vi "AddTagBusWebServiceToProject.vi"() -> ()   [LabVIEW 2013]
uses:
  <resource>/Framework/Providers/ws_project_provider/common/NI Web Service Provider.lvlib
panel:
  out "error out":errorcluster
  # "Please wait..."
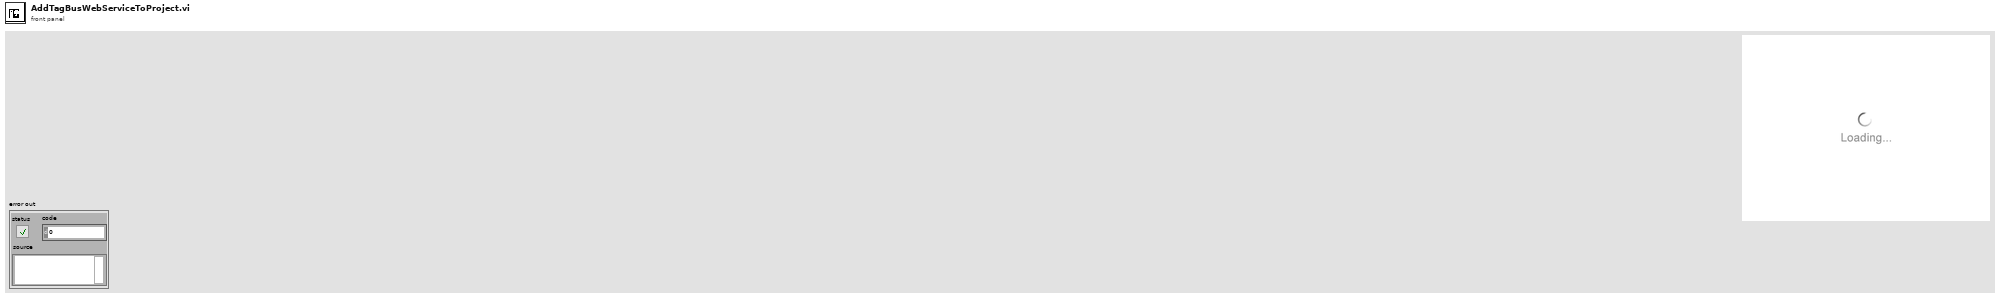
[diagram p1: front panel]
types:
  T1 = typedef "ws.ctl" = cluster{"Web Service":T2, "startup":path[], "wsmethods":path[], "private content":path[], "public content":path[], "wm ids":string[]}
  T2 = typedef "NI Web Service Provider.lvlib/Web Service.ctl" = cluster{"Name":string, "GUID":string, "Version":cluster{"Major":u16, "Minor":u16, "Fix":u16, "Build":u16}, "Serve index.html":bool, "Remote debugging":bool, "SSE2 optimizations":bool, "Exclusions":cluster{"Disconnect type definitions":bool, "Remove unused polymorphic VI instances":bool, "Remove unused members of project libraries":bool, "Modify project library file after removing unused members":bool}, "Disconnect inline subVIs":bool, "Auto-increment version":bool, "Web service VIs":T3[], "Static Permissions":string}
  T3 = typedef "NI Web Service Provider.lvlib/Web Service VI.ctl" = cluster{"item":u64, "item ID":string, "Web Service VI Type":T4, "Method":T5, "Load at startup":bool, "Keep in memory":bool, "Output type":T6, "Output format":T7, "Use headers":bool, "Buffered":bool, "Require API key":bool, "Permissions":string, "Standard URL":bool, "Include VI name in URL":bool, "Custom URL":string}
  T4 = typedef "NI Web Service Provider.lvlib/Web Service VI Type.ctl" = enum16{"<DUMMY>", "Web Method", "Auxiliary", "Internal", "Content"}
  T5 = typedef "NI Web Service Provider.lvlib/Web Service VI Method.ctl" = enum16{"<DUMMY>", "GET", "PUT", "POST", "DELETE", "OPTIONS", "HEAD", "TRACE"}
  T6 = typedef "NI Web Service Provider.lvlib/Web Service VI Output Type.ctl" = enum16{"Terminal", "Stream"}
  T7 = typedef "NI Web Service Provider.lvlib/Web Service VI Output Format.ctl" = enum16{"<DUMMY>", "Text", "XML", "HTML", "JSON"}
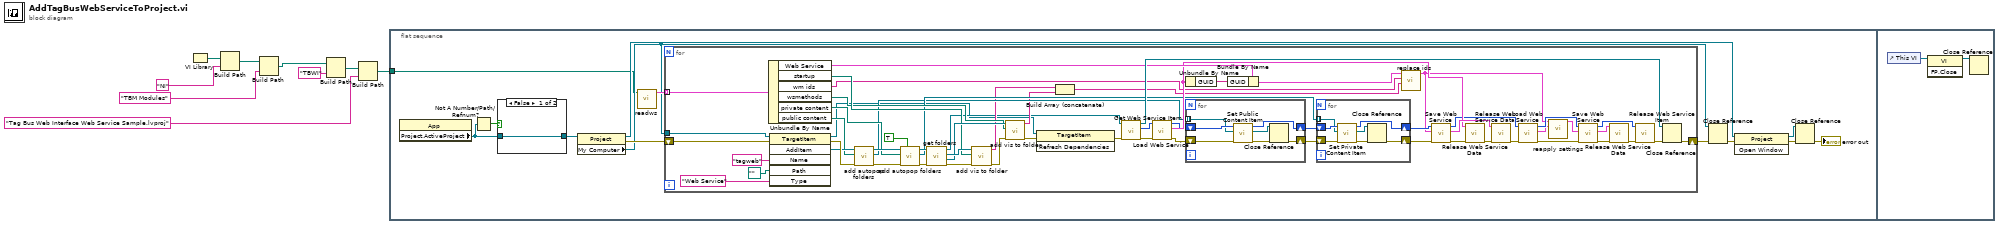
[diagram p0: block diagram]
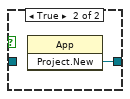
[diagram p2: hidden frame]
diagram:
  n1 = VI Library() -> (path=w5:path)
  n2 = Build Path(base path=w5, name or relative path="NI") -> (appended path=w7:path)
  n3 = Build Path(base path=w7, name or relative path="TBM Modules") -> (appended path=w4:path)
  n4 = Build Path(base path=w4, name or relative path="TBWI") -> (appended path=w3:path)
  n5 = Build Path(base path=w3, name or relative path="Tag Bus Web Interface Web Service Sample.lvproj") -> (appended path=w1:path)
  n6 = flat-sequence {
    tunnel: w1 -> [w10]
    frame #0 {
      n7 = property class="App"() -> ("Project.ActiveProject"=w13:refnum<vi>)  [unwired: 2 in, 2 out]
      n8 = Not A Number/Path/Refnum?(number/path/refnum=w13) -> (NaN/Path/Refnum?=w12:bool)
      n9 = case shown="False" w12 {
        tunnel: [w23 w24] -> w11
        tunnel: w13 -> [w23 _]
        frame False {
        }
        frame True {
          n10 = invoke class="App" method="Project.New"() -> ("Project:New"=w24:refnum<vi>)  [unwired: 3 in, 2 out]
        }
      }
      n11 = property class="Project"(reference=w11) -> (reference out=w19:refnum<vi>, error out=w21:errorcluster, "My Computer"=w15:refnum<vi>)  [unwired: 1 in]
      n12 = call "readws.vi"("Path"=w10) -> ("Array"=w22:T1[])  [unwired: 9 in, 1 out]
      n13 = for {
        tunnel: w22 -> [w66] mode=indexing
        shift-right: [w78] -> w14
        shift-left: w21 -> [w77]
        tunnel: w15 -> [w29]
        n14 = Unbundle By Name(w66) -> ("Web Service"=w61:T2, "startup"=w63:path[], "wm ids"=w44:string[], "wsmethods"=w62:path[], "private content"=w64:path[], "public content"=w65:path[])
        n15 = invoke class="TargetItem" method="AddItem"(reference=w29, error in=w77, "Name"="tagweb", "Path"=path "", "Type"="Web Service") -> (reference out=w25:refnum<vi>, error out=w76:errorcluster, "AddItem"=w75:refnum<vi>)  [unwired: 1 in, 3 out]
        n16 = call "add autopop folders.vi"("error in (no error)"=w76, "autopop"=w65, "ProjectItem in"=w75) -> ("error out"=w70:errorcluster, "items out"=w47:refnum<vi>[], "ProjectItem out"=w67:refnum<vi>)  [unwired: 6 in]
        n17 = call "add autopop folders.vi"("private?"=TRUE, "error in (no error)"=w70, "autopop"=w64, "ProjectItem in"=w67) -> ("error out"=w69:errorcluster, "items out"=w48:refnum<vi>[], "ProjectItem out"=w68:refnum<vi>)  [unwired: 5 in]
        n18 = call "get folders.vi"("error in"=w69, "web service in"=w68) -> ("error out"=w73:errorcluster, "web methods"=w72:refnum<vi>, "startup"=w74:refnum<vi>, "Web service project item out"=w26:refnum<vi>)  [unwired: 6 in]
        n19 = call "add vis to folder.vi"("error in"=w73, "startup"=w63, "ProjectItem in"=w74) -> ("error out"=w71:errorcluster, "ids"=w41:string[])  [unwired: 7 in]
        n20 = call "add vis to folder.vi"("error in"=w71, "startup"=w62, "ProjectItem in"=w72) -> ("error out"=w28:errorcluster, "ids"=w43:string[])  [unwired: 7 in]
        n21 = invoke class="TargetItem" method="Refresh Dependencies"(reference=w25, error in=w28) -> (error out=w27:errorcluster)  [unwired: 1 in, 2 out]
        n22 = Build Array (concatenate)(w41, w43) -> (w42:string[])
        n23 = call <resource>:"Get Web Service Item.vi"("Error In"=w27, "Web service project item"=w26) -> ("Error Out"=w59:errorcluster, "Web service item"=w60:u64, "Web service project item out"=w79:refnum<vi>)  [unwired: 7 in]
        n24 = call <resource>:"Load Web Service.vi"("Error In"=w59, "Web service item"=w60) -> ("Error Out"=w53:errorcluster, "Web Service"=w55:T2, "Web service item out"=w50:u64)  [unwired: 7 in]
        n25 = Unbundle By Name(w55) -> ("GUID"=w58:string)
        n26 = for {
          shift-right: [w92] -> w45
          shift-left: w53 -> [w95]
          shift-right: [w98] -> w51
          shift-left: w50 -> [w94]
          tunnel: w47 -> [w93] mode=indexing
          n27 = call <resource>:"Set Public Content Item.vi"("Error In"=w95, "Public content project item"=w93, "Web service item"=w94) -> ("Error Out"=w97:errorcluster, "Public content project item out"=w96:refnum<vi>, "Web service item out"=w98:u64)  [unwired: 6 in]
          n28 = Close Reference(reference=w96, error in (no error)=w97) -> (error out=w92:errorcluster)
        }
        n29 = Bundle By Name(cluster=w61, "GUID"=w58) -> (w46:T2)
        n30 = for {
          shift-right: [w91] -> w52
          shift-left: w45 -> [w86]
          shift-right: [w89] -> w49
          shift-left: w51 -> [w90]
          tunnel: w48 -> [w85] mode=indexing
          n31 = call <resource>:"Set Private Content Item.vi"("Error In"=w86, "Private content project item"=w85, "Web service item"=w90) -> ("Error Out"=w87:errorcluster, "Private content project item out"=w88:refnum<vi>, "Web service item out"=w89:u64)  [unwired: 6 in]
          n32 = Close Reference(reference=w88, error in (no error)=w87) -> (error out=w91:errorcluster)
        }
        n33 = call "replace ids.vi"("new ids"=w42, "old ids"=w44, "Web Service in"=w46) -> ("Web Service out"=w32:T2)  [unwired: 8 in]
        n34 = call <resource>:"Save Web Service.vi"("Error In"=w52, "Web Service"=w32, "Web service item"=w49) -> ("Error Out"=w57:errorcluster, "Web Service out"=w81:T2, "Web service item out"=w40:u64)  [unwired: 6 in]
        n35 = call <resource>:"Release Web Service Data.vi"("Error In"=w57, "Web Service"=w55) -> ("Error Out"=w56:errorcluster)  [unwired: 9 in]
        n36 = call <resource>:"Release Web Service Data.vi"("Error In"=w56, "Web Service"=w81) -> ("Error Out"=w39:errorcluster)  [unwired: 9 in]
        n37 = call <resource>:"Load Web Service.vi"("Error In"=w39, "Web service item"=w40) -> ("Error Out"=w33:errorcluster, "Web Service"=w30:T2, "Web service item out"=w35:u64)  [unwired: 7 in]
        n38 = call "reapply settings.vi"("ws settings in"=w30, "desired settings"=w32) -> ("ws settings out"=w31:T2)  [unwired: 9 in]
        n39 = call <resource>:"Save Web Service.vi"("Error In"=w33, "Web Service"=w31, "Web service item"=w35) -> ("Error Out"=w38:errorcluster, "Web Service out"=w34:T2, "Web service item out"=w36:u64)  [unwired: 6 in]
        n40 = call <resource>:"Release Web Service Data.vi"("Error In"=w38, "Web Service"=w34) -> ("Error Out"=w37:errorcluster)  [unwired: 9 in]
        n41 = call <resource>:"Release Web Service Item.vi"("Error In"=w37, "Web service item"=w36) -> ("Error Out"=w80:errorcluster)  [unwired: 9 in]
        n42 = Close Reference(reference=w79, error in (no error)=w80) -> (error out=w78:errorcluster)
      }
      n43 = Close Reference(reference=w15, error in (no error)=w14) -> (error out=w20:errorcluster)
      n44 = invoke class="Project" method="Open Window"(reference=w19, error in=w20) -> (reference out=w17:refnum<vi>, error out=w18:errorcluster)  [unwired: 1 in, 1 out]
      n45 = Close Reference(reference=w17, error in (no error)=w18) -> (error out=→"error out":errorcluster)
    }
    frame #1 {
      n46 = control-ref of="This VI"() -> (w100:refnum<vi>)
      n47 = invoke class="VI" method="FP.Close"(reference=w100) -> (reference out=w99:refnum<vi>)  [unwired: 2 in, 2 out]
      n48 = Close Reference(reference=w99) -> ()  [unwired: 1 in, 1 out]
    }
  }
